vi "Database Fetching.vi"() -> ()   [LabVIEW 2010]
doc: "This example fetches data from the specified table in a database named LabVIEW.mdb located in the LabVIEW examples>>database directory.\n\nThe table is assumed to be in the same format with the same datatypes as defined by the fetchdata table. You can use the Next and Previous buttons to move from the current record in the database table to the next or previous record."
uses:
  <vilib>/addons/database/Auxilliary.llb/DB Tools Cursor Type.ctl
  <vilib>/addons/database/_DB Variant To Data/Database Variant To Data.xnode
  <vilib>/addons/database/Connection.llb/DB Tools Open Connec (Path).vi
  <vilib>/addons/database/Connection.llb/Conn Execute.vi
  <vilib>/addons/database/Recordset.llb/Rec Get Recordset Properties (R).vi
  <vilib>/addons/database/Recordset.llb/Rec Destroy - Connection.vi
  <vilib>/addons/database/Recordset.llb/Rec Move To Previous Record (R).vi
  <vilib>/addons/database/Recordset.llb/Rec Move To Next Record (R).vi
  <vilib>/addons/database/Recordset.llb/Rec Fetch Integer Data (R).vi
  <vilib>/addons/database/Recordset.llb/Rec Fetch String Data (R).vi
  <vilib>/addons/database/Recordset.llb/Rec Fetch Binary Data (R).vi
  <vilib>/addons/database/NI_Database_API.lvlib
panel:
  out "record number":i32
  in  "stop":bool
  out "Phone Number":string
  out "Customer Number":i32
  out "Last Name":string
  out "First Name":string
  in  "previous \nrecord":bool
  in  "next\nrecord":bool
  # "INSTRUCTIONS:\n\nChoose the table from which to select data.  Run the VI.  Use the next record and previous record buttons to navigate the recordset. Press stop when finished."
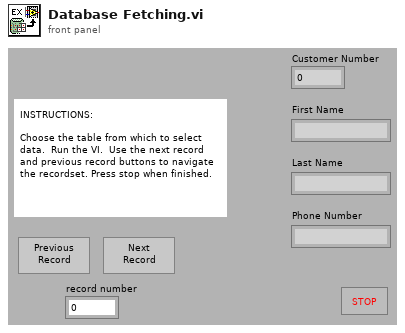
[diagram p1: front panel]
types:
  T1 = typedef "NI_Database_API.lvlib/DB Tools Cursor Type.ctl" = enum16{"forward-only", "keyset", "dynamic", "static"}
  T2 = typedef "NI_Database_API.lvlib/Conn ObjectReference.ctl" = refnum<k1>
  T3 = typedef "NI_Database_API.lvlib/Rec ObjectReference.ctl" = refnum<k1>
  T4 = typedef "NI_Database_API.lvlib/Rec Properties.ctl" = cluster{"column count":i32, "record index":i32, "record count":i32, "bof?":bool, "eof?":bool, "cursor type":T1, "cache size":i32, "state":enum16{"closed", "open"}}
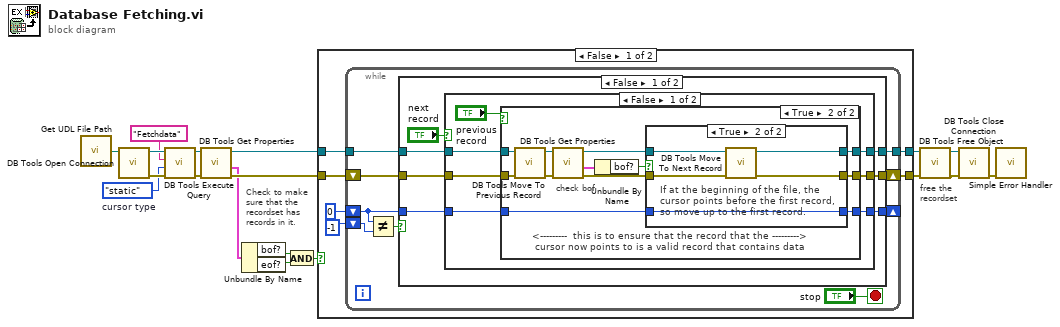
[diagram p0: block diagram]
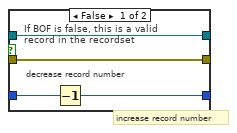
[diagram p3: hidden frame]
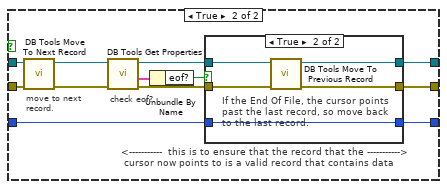
[diagram p4: hidden frame]
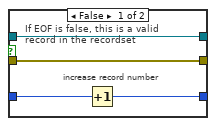
[diagram p5: hidden frame]
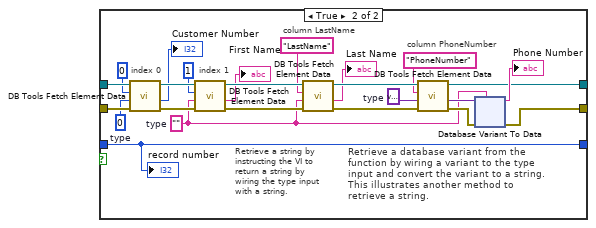
[diagram p6: hidden frame]
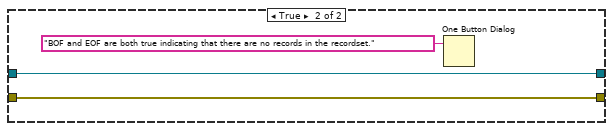
[diagram p7: hidden frame]
diagram:
  w15 = DB_Tools_Cursor_Type."static"  # cursor type
  # "free the\nrecordset"
  # "Check to make\nsure that the\nrecordset has\nrecords in it."
  n1 = call "Get UDL File Path.vi"() -> ("UDL file path"=w18:path)  [unwired: 1 in]
  n2 = call-poly <vilib>:"DB Tools Open Connection.vi"("connection information"=w18) -> ("error out"=w17:errorcluster, "connection reference"=w16:T2)  [unwired: 7 in]
  n3 = call-poly <vilib>:"DB Tools Execute Query.vi"("error in (no error)"=w17, "cursor type"=w15, "SQL query"="Fetchdata", "connection reference"=w16) -> ("error out"=w13:errorcluster, "recordset reference"=w14:T3)  [unwired: 4 in]
  n4 = call-poly <vilib>:"DB Tools Get Properties.vi"("error in (no error)"=w13, "recordset reference"=w14) -> ("error out"=w11:errorcluster, "recordset properties"=w10:T4, "recordset reference out"=w12:T3)  [unwired: 3 in]
  n5 = Unbundle By Name(w10) -> ("bof?"=w8:bool, "eof?"=w7:bool)
  n6 = And(x=w8, y=w7) -> (x .and. y?=w9:bool)
  n7 = case shown="False" w9 {
    tunnel: w12 -> [w24 w151]
    tunnel: w11 -> [w21 w150]
    tunnel: [w20 w151] -> w5
    tunnel: [w19 w150] -> w6
    frame False {
      n8 = while {
        tunnel: w24 -> [w33]
        shift-right: [w28] -> _
        shift-left: 0 -> [w30]
        shift-left: -1 -> [w31]
        shift-right: [w27] -> w19
        shift-left: w21 -> [w26]
        tunnel: [w25] -> w20
        stop <- "stop" stop-if-true
        n9 = Not Equal?(x=w30, y=w31) -> (x != y?=w29:bool)
        n10 = case shown="False" w29 {
          tunnel: w26 -> [w39 w116]
          tunnel: w33 -> [w38 w115]
          tunnel: w30 -> [w37 w96]
          tunnel: [w36 w96] -> w28
          tunnel: [w35 w94] -> w27
          tunnel: [w34 w95] -> w25
          frame False {
            n11 = case shown="False" "next\nrecord" {
              tunnel: w37 -> [w47 w79]
              tunnel: [w46 w78] -> w36
              tunnel: w39 -> [w44 w73]
              tunnel: [w45 w77] -> w35
              tunnel: w38 -> [w43 w74]
              tunnel: [w41 w72] -> w34
              frame False {
                n12 = case shown="True" "previous \nrecord" {
                  tunnel: w47 -> [w50 w54]
                  tunnel: [w50 w52] -> w46
                  tunnel: w44 -> [w49 w61]
                  tunnel: w43 -> [w48 w62]
                  tunnel: [w49 w55] -> w45
                  tunnel: [w48 w51] -> w41
                  frame False {
                  }
                  frame True {
                    # "<---------  this is to ensure that the record that the --------->\n cursor now points to is a valid record that contains data"
                    # "check bof"
                    n13 = call-poly <vilib>:"DB Tools Move To Previous Record.vi"("error in (no error)"=w61, "recordset reference"=w62) -> ("error out"=w60:errorcluster, "recordset reference out"=w59:T3)  [unwired: 8 in]
                    n14 = call-poly <vilib>:"DB Tools Get Properties.vi"("error in (no error)"=w60, "recordset reference"=w59) -> ("error out"=w57:errorcluster, "recordset properties"=w58:T4, "recordset reference out"=w56:T3)  [unwired: 3 in]
                    n15 = Unbundle By Name(w58) -> ("bof?"=w53:bool)
                    n16 = case shown="True" w53 {
                      tunnel: w56 -> [w63 w71]
                      tunnel: w57 -> [w64 w70]
                      tunnel: w54 -> [w66 w69]
                      tunnel: [w65 w69] -> w52
                      tunnel: [w64 w68] -> w55
                      tunnel: [w63 w67] -> w51
                      frame False {
                        # "If BOF is false, this is a valid record in the recordset"
                        # "decrease record number"
                        # "increase record number"
                        n17 = Decrement(x=w66) -> (x-1=w65:i32)
                      }
                      frame True {
                        # "If at the beginning of the file, the \ncursor points before the first record, \nso move up to the first record."
                        n18 = call-poly <vilib>:"DB Tools Move To Next Record.vi"("error in (no error)"=w70, "recordset reference"=w71) -> ("error out"=w68:errorcluster, "recordset reference out"=w67:T3)  [unwired: 8 in]
                      }
                    }
                  }
                }
              }
              frame True {
                # "<-----------  this is to ensure that the record that the ----------->\n cursor now points to is a valid record that contains data"
                # "check eof?"
                # "move to next\nrecord."
                n19 = call-poly <vilib>:"DB Tools Move To Next Record.vi"("error in (no error)"=w73, "recordset reference"=w74) -> ("error out"=w76:errorcluster, "recordset reference out"=w75:T3)  [unwired: 8 in]
                n20 = call-poly <vilib>:"DB Tools Get Properties.vi"("error in (no error)"=w76, "recordset reference"=w75) -> ("error out"=w80:errorcluster, "recordset properties"=w83:T4, "recordset reference out"=w81:T3)  [unwired: 3 in]
                n21 = Unbundle By Name(w83) -> ("eof?"=w82:bool)
                n22 = case shown="True" w82 {
                  tunnel: w81 -> [w84 w92]
                  tunnel: w80 -> [w85 w91]
                  tunnel: w79 -> [w87 w90]
                  tunnel: [w86 w90] -> w78
                  tunnel: [w85 w89] -> w77
                  tunnel: [w84 w88] -> w72
                  frame False {
                    # "If EOF is false, this is a valid record in the recordset"
                    # "increase record number"
                    n23 = Increment(x=w87) -> (x+1=w86:i32)
                  }
                  frame True {
                    # "If the End Of File, the cursor points\npast the last record, so move back \nto the last record."
                    n24 = call-poly <vilib>:"DB Tools Move To Previous Record.vi"("error in (no error)"=w91, "recordset reference"=w92) -> ("error out"=w89:errorcluster, "recordset reference out"=w88:T3)  [unwired: 8 in]
                  }
                }
              }
            }
          }
          frame True {
            w101 = 0  # type
            w104 = variant  # type
            w93 = ""  # type
            # "Retrieve a database variant from the\nfunction by wiring a variant to the type\ninput and convert the variant to a string.  \nThis illustrates another method to\nretrieve a string."
            # "Retrieve a string by \ninstructing the VI to \nreturn a string by \nwiring the type input \nwith a string."
            # "column PhoneNumber"
            # "column LastName"
            # "index 1"
            # "index 0"
            n25 = call-poly <vilib>:"DB Tools Fetch Element Data.vi"("error in (no error)"=w116, "type"=w101, "column index"=0, "recordset reference"=w115) -> ("error out"=w114:errorcluster, "data"=→"Customer Number":i32, "recordset reference out"=w113:T3)  [unwired: 3 in]
            n26 = call-poly <vilib>:"DB Tools Fetch Element Data.vi"("error in (no error)"=w114, "type"=w93, "column index"=1, "recordset reference"=w113) -> ("error out"=w112:errorcluster, "data"=→"First Name":string, "recordset reference out"=w111:T3)  [unwired: 3 in]
            n27 = call-poly <vilib>:"DB Tools Fetch Element Data.vi"("error in (no error)"=w112, "type"=w93, "column index"="LastName" ("SQL query"), "recordset reference"=w111) -> ("error out"=w110:errorcluster, "data"=→"Last Name":string, "recordset reference out"=w109:T3)  [unwired: 3 in]
            n28 = call-poly <vilib>:"DB Tools Fetch Element Data.vi"("error in (no error)"=w110, "type"=w104, "column index"="PhoneNumber" ("SQL query"), "recordset reference"=w109) -> ("error out"=w102:errorcluster, "data"=w103:variant, "recordset reference out"=w95:T3)  [unwired: 3 in]
            n29 = xnode "Database Variant To Data"("database variant"=w103, "error in"=w102, "type"=w93) -> ("data"=→"Phone Number":string, "error out"=w94:errorcluster)
            "record number" <- w96
          }
        }
      }
    }
    frame True {
      n30 = One Button Dialog(message="BOF and EOF are both true indicating that there are no records in the recordset.") -> ()  [unwired: 1 in, 1 out]
    }
  }
  n31 = call-poly <vilib>:"DB Tools Free Object.vi"("error in (no error)"=w6, "recordset reference"=w5) -> ("error out"=w3:errorcluster, "connection reference"=w4:T2)  [unwired: 8 in]
  n32 = call <vilib>:"DB Tools Close Connection.vi"("error in (no error)"=w3, "connection reference"=w4) -> ("error out"=w2:errorcluster)  [unwired: 5 in]
  n33 = call <vilib>:"Simple Error Handler.vi"("error in (no error)"=w2) -> ()  [unwired: 4 in, 5 out]
